vi "Periodic Tasks.vi"(8 "error in":errorcluster) -> ()   [LabVIEW 2013]
doc: "This VI runs in parallel to other tasks. It can contain as many user-defined periodic loops as you need. These can carry out PID or other sorts of timed response."
uses:
  Program Files (x86)/National Instruments/LabVIEW 2013/examples/FRC/I2C/ADXL345 I2C/Driver/ADXL345 I2C Axis.ctl
  <vilib>/Rock Robotics/SystemInterfaces/Utilities/FPGA_UtilitiesLED Source.ctl
  <vilib>/Rock Robotics/SystemInterfaces/Utilities/FPGA_UtilitiesLED State.ctl
  Robot Global Data.vi
  <vilib>/Rock Robotics/WPI/RobotDrive/WPI_RobotDriveGetSetRefNum.vi
  <vilib>/Rock Robotics/WPI/Joystick/WPI_JoystickGetSetRefNum.vi
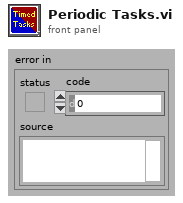
[diagram p1: front panel]
types:
  T1 = typedef "WPI_JoystickDevRef.ctl" = cluster{"Device":T2}
  T2 = typedef "WPI_JoystickDeviceEnum.ctl" = enum16{"USB 1", "USB 2", "USB 3", "USB 4", "Kinect 1", "Kinect 2"}
  T3 = typedef "WPI_RobotDriveDevRef.ctl" = cluster{"DevStatus":errorcluster, "Motors[]":T4[], "Square Inputs":bool, "Max Output":dbl, "Isochronous":bool}
  T4 = typedef "WPI_MotorControlDeviceRef.ctl" = cluster{"DeviceStatus":errorcluster, "Type":enum16{"PWM", "CAN"}, "PWM":cluster{"Digital Module":T5, "PWM Channel":T6, "DeadBand":T7}, "CAN":cluster{"Device Number":u8, "Control Mode":T8, "Semaphore":T9, "Max Vout":dbl}, "Invert":bool, "TransformRef":T10, "InvTransformRef":T10}
  T5 = typedef "FPGA_TypedefDigitalModule.ctl" = enum16{"Digital Module 1", "Digital Module 2"}
  T6 = typedef "FPGA_DIOPWMChannel.ctl" = enum8{"PWM 1", "PWM 2", "PWM 3", "PWM 4", "PWM 5", "PWM 6", "PWM 7", "PWM 8", "PWM 9", "PWM 10", "Invalid"}
  T7 = typedef "WPI_PWMDeadband.ctl" = cluster{"Name":string, "maxPositivePwm":i32, "minPositivePwm":i32, "centerPwm":i32, "maxNegativePwm":i32, "minNegativePwm":i32, "angularRange":u16}
  T8 = typedef "WPI_CANJaguar_ControlMode.ctl" = enum8{"Percent VBus", "Current", "Speed", "Position", "Voltage"}
  T9 = typedef "Semaphore RefNum" = refnum<k1>
  T10 = typedef "WPI_PWMTransform_ConPane.ctl" = refnum<vi>
  T11 = cluster{"JoystickDevRef":T1, "RobotDriveDevRef":T3}
  T12 = typedef "WPI_GyroDevRef.ctl" = cluster{"DevStatus":errorcluster, "Analog Module":T13, "Analog Channel":T14, "Offset":dbl, "Gain (VoltsPerDegree/Second)":dbl}
  T13 = typedef "FPGA_TypedefAnalogModule.ctl" = enum16{"Analog Module 1", "Analog Module 2"}
  T14 = typedef "FPGA_AIChannel.ctl" = enum8{"AI 1", "AI 2", "AI 3", "AI 4", "AI 5", "AI 6", "AI 7", "AI 8", "Invalid"}
  T15 = typedef "WPI_I2CDevRef.ctl" = cluster{"DevStatus":errorcluster, "Digital Module":T5, "Device Address":u8}
  T16 = typedef "WPI_EncoderDevRef.ctl" = cluster{"DevStatus":errorcluster, "EncoderIndex":T17, "CounterIndex":T18, "DistancePerCount":dbl, "Decoding Type":T19}
  T17 = typedef "FPGA_EncoderIdx.ctl" = enum8{"Enc 0", "Enc 1", "Enc 2", "Enc 3", "Invalid"}
  T18 = typedef "FPGA_CounterCtrSystemIndex.ctl" = enum8{"Ctr 0", "Ctr 1", "Ctr 2", "Ctr 3", "Ctr 4", "Ctr 5", "Ctr 6", "Ctr 7", "Invalid"}
  T19 = typedef "WPI_EncoderType.ctl" = enum16{"1x", "2x", "4x"}
  T20 = typedef "ADXL345 I2C Axis.ctl" = u8
  T21 = cluster{" Rate":dbl, "Current angle":dbl, "Revolutions":dbl, "Distance":dbl, "Reset":bool}
  T22 = typedef "FPGA_UtilitiesLED State.ctl" = enum16{"Off", "On", "Toggle"}
  T23 = typedef "FPGA_UtilitiesLED Source.ctl" = enum16{"User LED", "FPGA LED"}
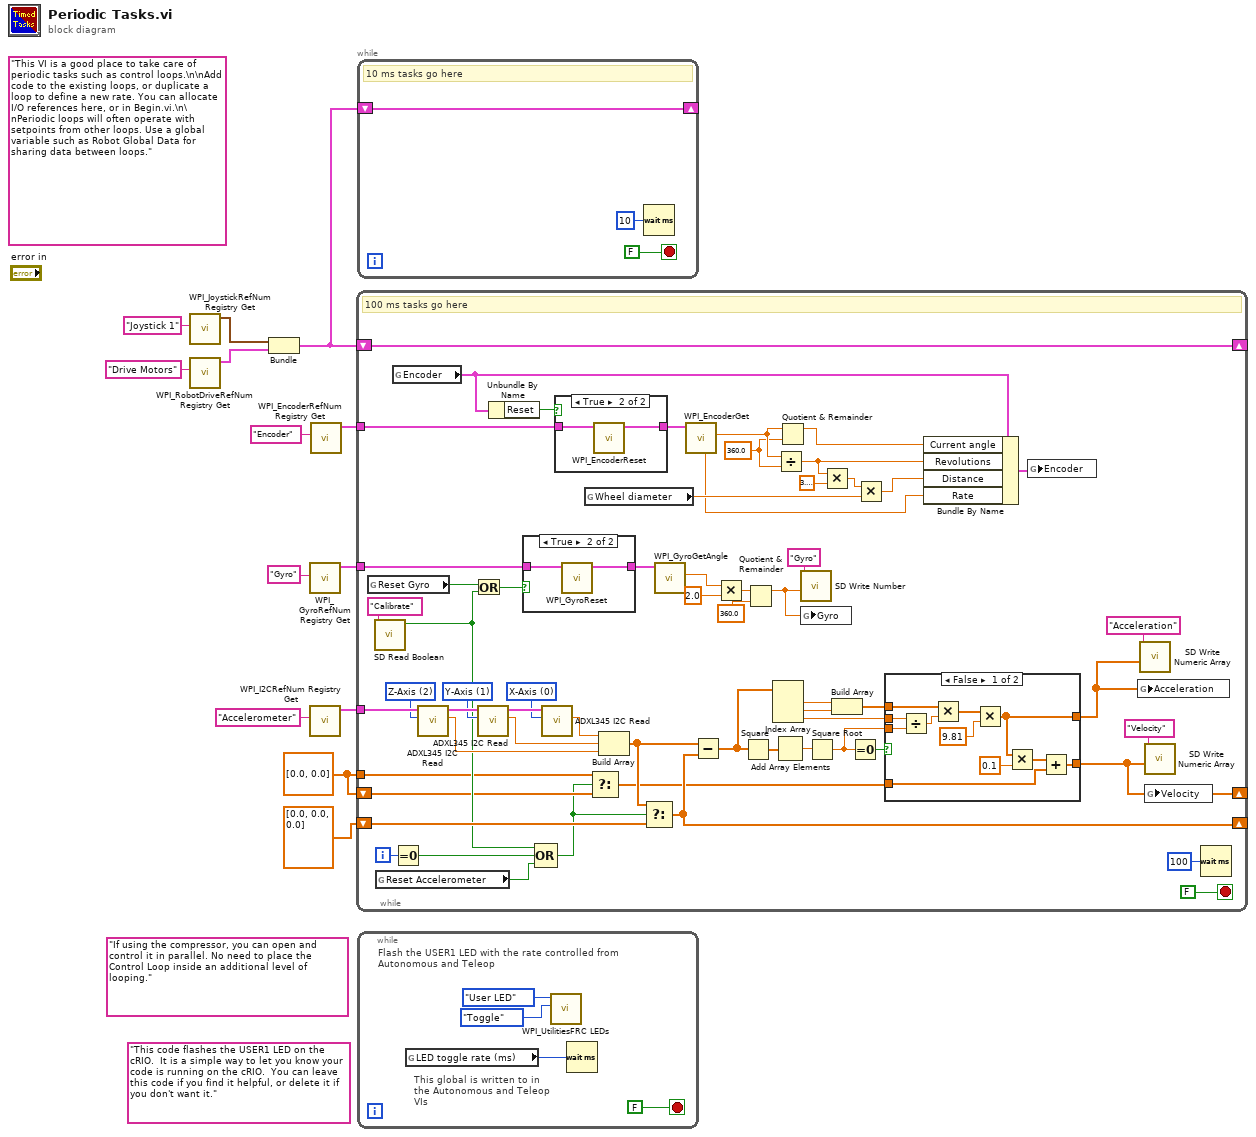
[diagram p0: block diagram]
diagram:
  w4 = dbl[] [0.0, 0.0] ("f")
  (unwired) "If using the compressor, you can open and control it in parallel. No need to place the Control Loop inside an additional level of looping."
  (unwired) "This code flashes the USER1 LED on the cRIO.  It is a simple way to let you know your code is running on the cRIO.  You can leave this code if you find it helpful, or delete it if you don't want it."
  (unwired) "This VI is a good place to take care of periodic tasks such as control loops.\n\nAdd code to the existing loops, or duplicate a loop to define a new rate. You can allocate I/O references here, or in Begin.vi.\n\nPeriodic loops will often operate with setpoints from other loops. Use a global variable such as Robot Global Data for sharing data between loops."
  n1 = call <vilib>:"WPI_JoystickRefNum Registry Get.vi"("refnum name"="Joystick 1") -> ("JoystickDevRef"=w11:T1)  [unwired: 1 in, 9 out]
  n2 = call <vilib>:"WPI_RobotDriveRefNum Registry Get.vi"("refnum name"="Drive Motors") -> ("RobotDriveDevRef"=w10:T3)  [unwired: 1 in, 9 out]
  n3 = Bundle("JoystickDevRef"=w11, "RobotDriveDevRef"=w10) -> (w9:T11)  [unwired: 1 out]
  n4 = call <vilib>:"WPI_GyroRefNum Registry Get.vi"("refnum name"="Gyro") -> ("GyroDevRef"=w7:T12)  [unwired: 9 in, 1 out]
  n5 = call <vilib>:"WPI_I2CRefNum Registry Get.vi"("refnum name"="Accelerometer") -> ("I2CDevRef"=w6:T15)  [unwired: 9 in, 1 out]
  n6 = call <vilib>:"WPI_EncoderRefNum Registry Get.vi"("refnum name"="Encoder") -> ("EncoderDevRef"=w2:T16)  [unwired: 9 in, 1 out]
  n7 = while {
    shift-right: [w72] -> _
    shift-left: w9 -> [w72]
    tunnel: w6 -> [w69]
    tunnel: w7 -> [w63]
    shift-right: [w55] -> _
    shift-left: dbl[] [0.0, 0.0, 0.0] ("f") -> [w53]
    tunnel: w4 -> [w37]
    shift-right: [w29] -> _
    shift-left: w4 -> [w36]
    tunnel: w2 -> [w16]
    i -> [w54]
    stop <- FALSE stop-if-true
    w24 = 360.0 ("y")
    w59 = T20 0 items=["X-Axis", "Y-Axis", "Z-Axis"] ("Axis")
    w70 = T20 1 items=["X-Axis", "Y-Axis", "Z-Axis"] ("Axis")
    w62 = T20 2 items=["X-Axis", "Y-Axis", "Z-Axis"] ("Axis")
    # "100 ms tasks go here"
    n8 = global read "Robot Global Data.vi" "Reset Gyro"() -> (w44:bool)
    n9 = call <vilib>:"SD Read Boolean.vi"("Name"="Calibrate") -> ("Boolean"=w41:bool)  [unwired: 8 in, 2 out]
    n10 = global read "Robot Global Data.vi" "Reset Accelerometer"() -> (w42:bool)
    n11 = global read "Robot Global Data.vi" "Encoder"() -> (w15:T21)
    n12 = Equal To 0?(x=w54) -> (x = 0?=w43:bool)
    n13 = call "ADXL345 I2C Read.vi"("Axis"=w62, "I2CDevRef"=w69) -> ("Acceleration"=w45:dbl, "I2CDevRef Out"=w71:T15)  [unwired: 1 in, 7 out]
    n14 = Or(x=w44, y=w41) -> (x .or. y?=w58:bool)
    n15 = call "ADXL345 I2C Read.vi"("Axis"=w70, "I2CDevRef"=w71) -> ("Acceleration"=w49:dbl, "I2CDevRef Out"=w60:T15)  [unwired: 1 in, 7 out]
    n16 = Unbundle By Name(w15) -> ("Reset"=w17:bool)
    n17 = case shown="True" w58 {
      tunnel: w63 -> [w91 w93]
      tunnel: [w91 w92] -> w68
      frame False {
      }
      frame True {
        n18 = call <vilib>:"WPI_GyroReset.vi"("GyroDevRef"=w93) -> ("GyroDevRef"=w92:T12)  [unwired: 9 in, 1 out]
      }
    }
    n19 = Compound Arithmetic op=OR(w41, w43, w42) -> (w35:bool)
    n20 = call "ADXL345 I2C Read.vi"("Axis"=w59, "I2CDevRef"=w60) -> ("Acceleration"=w50:dbl)  [unwired: 1 in, 8 out]
    n21 = case shown="True" w17 {
      tunnel: [w75 w77] -> w27
      tunnel: w16 -> [w75 w76]
      frame False {
      }
      frame True {
        n22 = call <vilib>:"WPI_EncoderReset.vi"("EncoderDevRef"=w76) -> ("EncoderDevRef"=w77:T16)  [unwired: 1 in, 9 out]
      }
    }
    n23 = global read "Robot Global Data.vi" "Wheel diameter"() -> (w22:dbl)
    n24 = Select(t=w37, s=w35, f=w36) -> (s? t:f=w28:dbl[])
    n25 = Build Array(w50, w49, w45) -> (w56:dbl[])
    n26 = Select(t=w56, s=w35, f=w53) -> (s? t:f=w55:dbl[])
    n27 = call <vilib>:"WPI_GyroGetAngle.vi"("GyroDevRef"=w68) -> ("Angle"=w67:dbl)  [unwired: 7 in, 3 out]
    n28 = call <vilib>:"WPI_EncoderGet.vi"("EncoderDevRef"=w27) -> ("Distance"=w26:dbl, "Rate"=w18:dbl)  [unwired: 5 in, 4 out]
    n29 = Subtract(x=w56, y=w55) -> (x-y=w40:dbl[])
    n30 = Multiply(x=w67, y=2.0) -> (x*y=w65:dbl)
    n31 = Square(x=w40) -> (x^2=w51:dbl[])
    n32 = Quotient & Remainder(x=w65, y=360.0) -> (x-y*floor(x/y)=w57:dbl)  [unwired: 1 out]
    n33 = Index Array(array=w40) -> (element #1=w39:dbl, element #2=w38:dbl, element #3=w31:dbl)  [unwired: 3 in]
    n34 = Add Array Elements(numeric array=w51) -> (sum=w52:dbl)
    n35 = Divide(x=w26, y=w24) -> (x/y=w20:dbl)
    n36 = Quotient & Remainder(x=w26, y=w24) -> (x-y*floor(x/y)=w19:dbl)  [unwired: 1 out]
    n37 = call <vilib>:"SD Write Number.vi"("Numeric"=w57, "Name"="Gyro") -> ()  [unwired: 8 in, 2 out]
    n38 = global write "Robot Global Data.vi" "Gyro"(w57) -> ()
    n39 = Square Root(x=w52) -> (sqrt(x)=w33:dbl)
    n40 = Multiply(x=w20, y=3.141592653589793) -> (x*y=w23:dbl)
    n41 = Build Array(w39, w38) -> (w32:dbl[])
    n42 = Equal To 0?(x=w33) -> (x = 0?=w34:bool)
    n43 = Multiply(x=w23, y=w22) -> (x*y=w21:dbl)
    n44 = case shown="False" w34 {
      tunnel: w32 -> [w87 w90]
      tunnel: w33 -> [w88 _]
      tunnel: w31 -> [w86 _]
      tunnel: [w80 w90] -> w30
      tunnel: [w79 w89] -> w29
      tunnel: w28 -> [w78 w89]
      frame False {
        n45 = Divide(x=w86, y=w88) -> (x/y=w85:dbl)
        n46 = Multiply(x=w87, y=w85) -> (x*y=w84:dbl[])
        n47 = Multiply(x=w84, y=9.81) -> (x*y=w80:dbl[])
        n48 = Multiply(x=w80, y=0.1) -> (x*y=w81:dbl[])
        n49 = Add(x=w81, y=w78) -> (x+y=w79:dbl[])
      }
      frame True {
      }
    }
    n50 = Bundle By Name(cluster=w15, "Current angle"=w19, "Revolutions"=w20, "Distance"=w21, "Rate"=w18) -> (w14:T21)
    n51 = global write "Robot Global Data.vi" "Encoder"(w14) -> ()
    n52 = global write "Robot Global Data.vi" "Acceleration"(w30) -> ()
    n53 = call <vilib>:"SD Write Numeric Array.vi"("Numeric Array"=w30, "Name"="Acceleration") -> ()  [unwired: 8 in, 2 out]
    n54 = call <vilib>:"SD Write Numeric Array.vi"("Numeric Array"=w29, "Name"="Velocity") -> ()  [unwired: 8 in, 2 out]
    n55 = global write "Robot Global Data.vi" "Velocity"(w29) -> ()
    n56 = Wait (ms)(milliseconds to wait=u32 100) -> ()  [unwired: 1 out]
  }
  n57 = while {
    shift-right: [w94] -> _
    shift-left: w9 -> [w94]
    stop <- FALSE stop-if-true
    # "10 ms tasks go here"
    n58 = Wait (ms)(milliseconds to wait=u32 10) -> ()  [unwired: 1 out]
  }
  n59 = while {
    stop <- FALSE stop-if-true
    # "This global is written to in the Autonomous and Teleop VIs"
    # "Flash the USER1 LED with the rate controlled from Autonomous and Teleop"
    n60 = global read "Robot Global Data.vi" "LED toggle rate (ms)"() -> (w97:u32)
    n61 = call <vilib>:"WPI_UtilitiesFRC LEDs.vi"("State"=FPGA_UtilitiesLED_State."Toggle", "LED Type"=FPGA_UtilitiesLED_Source."User LED") -> ()  [unwired: 1 in, 9 out]
    n62 = Wait (ms)(milliseconds to wait=w97) -> ()  [unwired: 1 out]
  }
